vi "Actor Core.vi"(8 "error in":errorcluster, 11 "Root Panel Actor in":refnum<class "Root Panel Actor.lvclass">) -> (0 "error out":errorcluster, 3 "Actor out":refnum<class "Actor.lvclass">)   [LabVIEW 2021, in "Root Panel.lvlib" / "Root Panel Actor.lvclass"]
doc: "The user interface for this panel.\n\n----\nPlease see the following web address for additional documentation and tutorial information:\nhttp://www.mooregoodideas.com/mgi-panel-manager/\n\nAuthor: Derek Trepanier\n\nCopyright (c) 2018, Moore Good Ideas, Inc.\n\nAll rights reserved.\n\nRedistribution and use in source and binary forms, with or without modification, are permitted provided that the following conditions are met:\n\n * Redistributions of source code must retain the above copyright notice, this list of conditions and the following disclaimer.\n * Redistributions in binary form must reproduce the above copyright notice, this list of conditions and the following disclaimer in the documentation and/or other materials provided with the distribution.\n * Neither the name of Moore Good Ideas, Inc. nor the names of its contributors may be used to endorse or promote products derived from this software without specific prior written permission.\n\nTHIS SOFTWARE IS PROVIDED BY THE COPYRIGHT HOLDERS AND CONTRIBUTORS \"AS IS\" AND ANY EXPRESS OR IMPLIED WARRANTIES, INCLUDING, BUT NOT LIMITED TO, THE IMPLIED WARRANTIES OF MERCHANTABILITY AND FITNESS FOR A PARTICULAR PURPOSE ARE DISCLAIMED. IN NO EVENT SHALL THE COPYRIGHT OWNER OR CONTRIBUTORS BE LIABLE FOR ANY DIRECT, INDIRECT, INCIDENTAL, SPECIAL, EXEMPLARY, OR CONSEQUENTIAL DAMAGES (INCLUDING, BUT NOT LIMITED TO, PROCUREMENT OF SUBSTITUTE GOODS OR SERVICES; LOSS OF USE, DATA, OR PROFITS; OR BUSINESS INTERRUPTION) HOWEVER CAUSED AND ON ANY THEORY OF LIABILITY, WHETHER IN CONTRACT, STRICT LIABILITY, OR TORT (INCLUDING NEGLIGENCE OR OTHERWISE) ARISING IN ANY WAY OUT OF THE USE OF THIS SOFTWARE, EVEN IF ADVISED OF THE POSSIBILITY OF SUCH DAMAGE."
uses:
  Root Panel Actor.lvclass
  C:/Program Files (x86)/National Instruments/LabVIEW 2021/vi.lib/MGI/Panel Manager/Panel Actor/Panel Actor/Panel Actor.lvclass
  <vilib>/ActorFramework/Actor/Actor.lvclass
  Root Panel Actor.lvclass/Root Panel Actor.ctl
  <vilib>/ActorFramework/Message Enqueuer/Message Enqueuer.lvclass/Message Enqueuer.ctl
  <vilib>/ActorFramework/Message Enqueuer/Enqueue.vi
  <vilib>/ActorFramework/Stop Msg/Stop Msg.lvclass
  C:/Program Files (x86)/National Instruments/LabVIEW 2021/vi.lib/ActorFramework/Message/Message.lvclass
  Appearance Actor/Appearance Actor Messages/UI Event-Close-Value Change Msg/UI Event-Close-Value Change Msg.lvclass
  Appearance Actor/Appearance Actor Messages/UI Event-Maximize-Value Change Msg/UI Event-Maximize-Value Change Msg.lvclass
  Appearance Actor/Appearance Actor Messages/UI Event-Minimize-Value Change Msg/UI Event-Minimize-Value Change Msg.lvclass
  Appearance Actor/Appearance Actor Messages/UI Event-Settings-Value Change Msg/UI Event-Settings-Value Change Msg.lvclass
  Appearance Actor/Appearance Actor Messages/UI Event-Title Bar-Mouse Down Msg/UI Event-Title Bar-Mouse Down Msg.lvclass
  <vilib>/ActorFramework/Message Priority Queue/Priority Enqueue.vi
  Appearance Actor/Appearance Actor/Appearance Actor.lvclass
  <vilib>/MGI/Panel Manager/Panel Actor/Panel Actor/Panel Actor.lvclass
  <vilib>/MGI/Panel Manager/Panel Actor/Panel Actor Messages/Show Panel Msg/Show Panel Msg.lvclass
  <vilib>/Thomas ALLIBE/Path Utilities/Path Utilities.lvlib
panel:
  in  "Title Bar L":bool
  out "App Icon":picture
  in  "Title Bar M":bool
  out "TB.Title":string
  in  "Dark-TB.Button.Maximize":bool
  in  "Light-TB.Button.Maximize":bool
  in  "Dark-TB.CloseButton":bool
  in  "Light-TB.CloseButton":bool
  in  "Dark-TB.Button.Minimize":bool
  in  "Light-TB.Button.Minimize":bool
  in  "Title Bar R":bool
  in  "Dark-SM.Button.Settings":bool
  in  "Light-SM.Button.Settings":bool
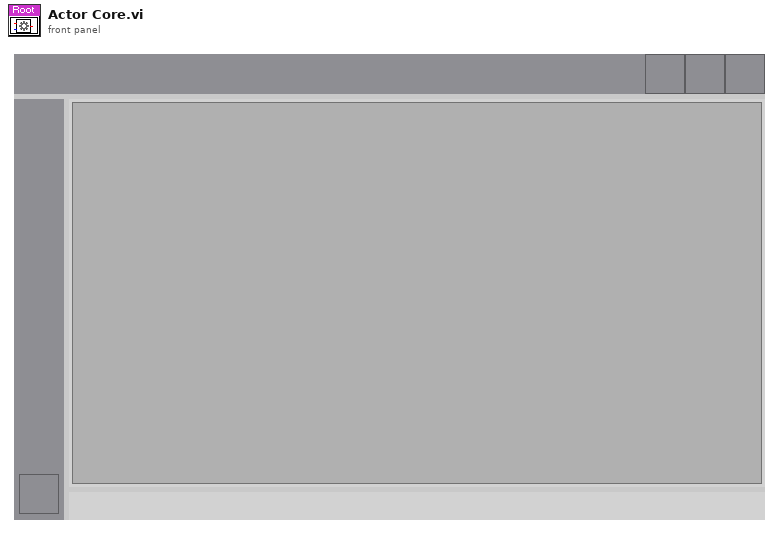
[diagram p1: front panel]
types:
  T1 = cluster{"left":i16, "top":i16, "right":i16, "bottom":i16}
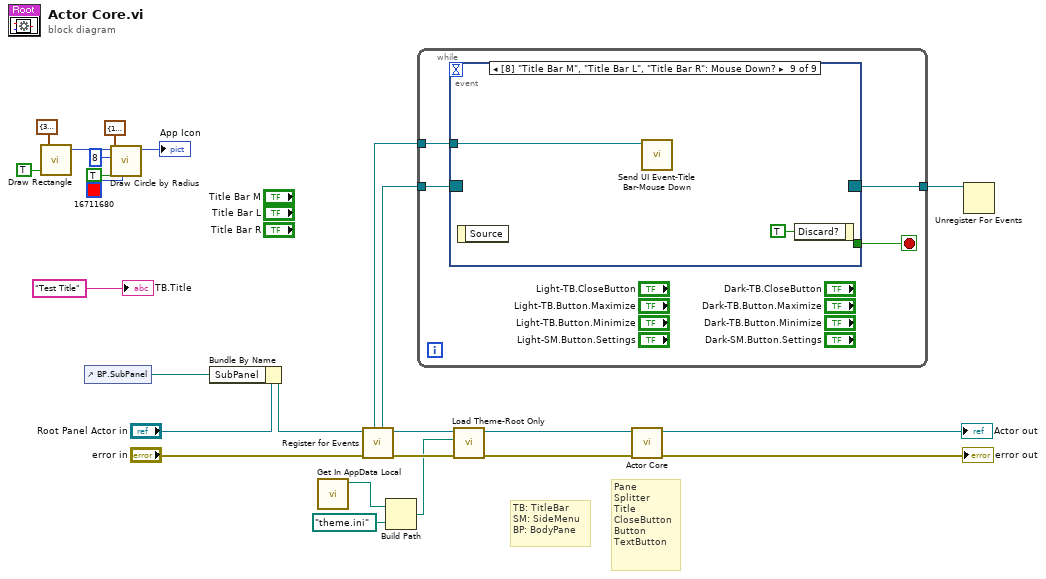
[diagram p0: block diagram]
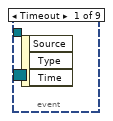
[diagram p2: hidden frame]
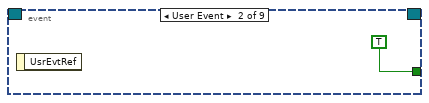
[diagram p3: hidden frame]
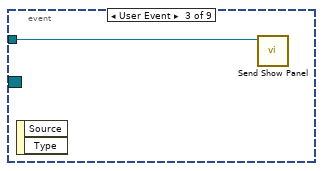
[diagram p4: hidden frame]
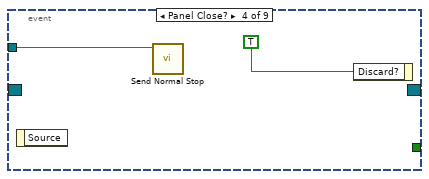
[diagram p5: hidden frame]
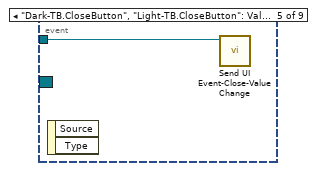
[diagram p6: hidden frame]
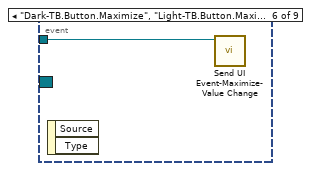
[diagram p7: hidden frame]
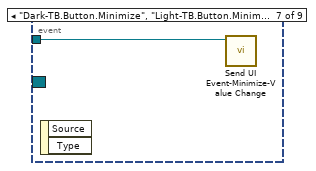
[diagram p8: hidden frame]
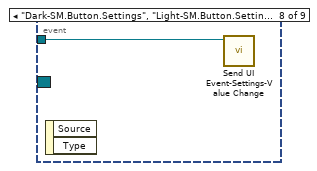
[diagram p9: hidden frame]
diagram:
  # "Pane\nSplitter\nTitle\nCloseButton\nButton\nTextButton"
  # "TB: TitleBar\nSM: SideMenu\nBP: BodyPane"
  n1 = call <vilib>:"Draw Rectangle.vi"("rect"=T1 {"left"=3, "top"=3, "right"=40, "bottom"=30}, "fill?(F)"=TRUE) -> ("new picture"=w19:picture)  [unwired: 7 in]
  n2 = control-ref of="BP.SubPanel"() -> (w1:refnum<vi>)
  n3 = call <vilib>:"Draw Circle by Radius.vi"("color(black)"=u32 16711680, "fill?(F)"=TRUE, "pixel center"=cluster{"horizontal":i16, "vertical":i16} {"horizontal"=15, "vertical"=12}, "radius"=i16 8, "picture"=w19) -> ("new picture"=→"App Icon":picture)  [unwired: 6 in]
  n4 = Bundle By Name(cluster="Root Panel Actor in", "SubPanel"=w1) -> (w4:refnum<class "Root Panel Actor.lvclass">)
  n5 = call <vilib>:"Get In AppData Local.vi"() -> ("Path"=w9:path)  [unwired: 10 in, 1 out]
  n6 = call <vilib>:"Register for Events.vi"("Error In"="error in", "Panel Actor in"=w4) -> ("Error Out"=w11:errorcluster, "Panel Actor out"=w12:refnum<class "Root Panel Actor.lvclass">, "Pnl Actor"=w22:refnum<event-registration>, "Self Enqueuer"=w23:refnum<class "Message Enqueuer.lvclass">)  [unwired: 6 in]
  n7 = Build Path(base path=w9, name or relative path=path "theme.ini") -> (appended path=w7:path)
  n8 = while {
    tunnel: w22 -> [w29]
    tunnel: w23 -> [w28]
    tunnel: [w26] -> w24
    stop <- w27 stop-if-true
    n9 = event shown="[8] \"Title Bar M\", \"Title Bar L\", \"Title Bar R\": Mouse Down?" {
      selector: w29 -> [_ _ _ _ _ _ _ _ _]
      dyn-events: [_ _ _ _ _ _ _ _ _] -> w26
      timeout: _ -> [_ _ _ _ _ _ _ _ _]
      tunnel: w28 -> [_ _ w31 w33 w34 w35 w36 w37 w38]
      tunnel: [_ TRUE _ _ _ _ _ _ _] -> w27
      event Timeout {
        n10 = event-data() -> ()  [unwired: 1 in, 3 out]
      }
      event User Event {
        n11 = event-data() -> ()  [unwired: 1 in, 1 out]
      }
      event User Event {
        n12 = event-data() -> ()  [unwired: 1 in, 2 out]
        n13 = call <vilib>:"Send Show Panel.vi"("Message Enqueuer in"=w31) -> ()  [unwired: 9 in, 2 out]
      }
      event Panel Close? {
        n14 = event-data() -> ()  [unwired: 1 in, 1 out]
        n15 = call <vilib>:"Send Normal Stop.vi"("Message Enqueuer"=w33) -> ()  [unwired: 10 in, 1 out]
        n16 = event-data("Discard?"=TRUE) -> ()  [unwired: 1 in, 1 out]
      }
      event "Dark-TB.CloseButton", "Light-TB.CloseButton": Value Change {
        n17 = event-data() -> ()  [unwired: 1 in, 2 out]
        n18 = call "Send UI Event-Close-Value Change.vi"("Message Enqueuer"=w34) -> ()  [unwired: 9 in, 2 out]
      }
      event "Dark-TB.Button.Maximize", "Light-TB.Button.Maximize": Value Change {
        n19 = event-data() -> ()  [unwired: 1 in, 2 out]
        n20 = call "Send UI Event-Maximize-Value Change.vi"("Message Enqueuer"=w35) -> ()  [unwired: 9 in, 2 out]
      }
      event "Dark-TB.Button.Minimize", "Light-TB.Button.Minimize": Value Change {
        n21 = event-data() -> ()  [unwired: 1 in, 2 out]
        n22 = call "Send UI Event-Minimize-Value Change.vi"("Message Enqueuer"=w36) -> ()  [unwired: 9 in, 2 out]
      }
      event "Dark-SM.Button.Settings", "Light-SM.Button.Settings": Value Change {
        n23 = event-data() -> ()  [unwired: 1 in, 2 out]
        n24 = call "Send UI Event-Settings-Value Change.vi"("Message Enqueuer"=w37) -> ()  [unwired: 9 in, 2 out]
      }
      event "Title Bar M", "Title Bar L", "Title Bar R": Mouse Down? {
        n25 = event-data() -> ()  [unwired: 1 in, 1 out]
        n26 = call "Send UI Event-Title Bar-Mouse Down.vi"("Message Enqueuer"=w38) -> ()  [unwired: 9 in, 2 out]
        n27 = event-data("Discard?"=TRUE) -> ()  [unwired: 1 in, 1 out]
      }
    }
  }
  n28 = call-dynamic "Load Theme-Root Only.vi"("Error In"=w11, "Theme File Path"=w7, "Appearance Actor in"=w12) -> ("Error Out"=w6:errorcluster, "Appearance Actor out"=w10:refnum<class "Root Panel Actor.lvclass">)  [unwired: 7 in]
  n29 = call-parent "Actor Core.vi"("error in"=w6, "Appearance Actor in"=w10) -> ("error out"=→"error out":errorcluster, "Actor out"=→"Actor out":refnum<class "Actor.lvclass">)  [unwired: 8 in]
  n30 = Unregister For Events(event registration refnum=w24) -> ()  [unwired: 1 in, 1 out]
  "TB.Title" <- "Test Title" ("Title")
